vi "Choreo_Choreo_LoadTrajectoryType.vi"(11 "FileName":string="C:\\Users\\Jim\\Desktop\\PathPlanner24\\Choreo\\ChoreoTest.TRAJ") -> (0 "error out":errorcluster, 3 "TrajectoryType":T1, 4 "Full Filename":string)   [LabVIEW 2019, in "ChoreoLib.lvlib"]
doc: "Determine the type of trajectory of a file in the deploy directory. Choreolib expects .traj files to be placed in /deploy/choreo/<trajectoryName>.traj.\n\nInputs: \n - filename - string - The name of the trajectory file. See notes below on file naming.\n\nOutputs:\n - TrajectoryType - enum - Type of trajectory found in the file.\n - Error out - cluster - Error cluster\n - Full Filename - string - fully qualified file name.\n\nNotes on file naming:\n - The file does not need to include the \".traj\" extension. This is added if not present.\n - The file name can be a simple file or an absolute path. If a simple file name is used the default path on the RoboRIO is: \"home:\\lvuser\\natinst\\LabVIEW Data\\choreo\". On a Windows PC the default path is the LabVIEW default directory\\choreo. Normally this is: “%HOMEDRIVE%%HOMEPATH%\\Documents\\LabView Data\\choreo\".\n - Filenames on the RoboRIO, which runs Linux, are case sensitive."
uses:
  ChoreoLib.lvlib
  ENum/Choreo_Util_TrajectoryType.ctl
panel:
  in  "error in (no error)":errorcluster
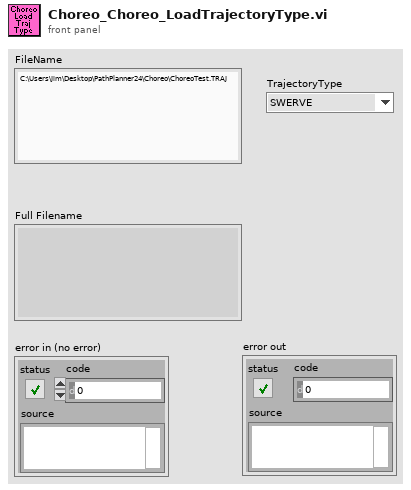
[diagram p1: front panel]
types:
  T1 = typedef "ChoreoLib.lvlib/Choreo_Util_TrajectoryType.ctl" = enum16{"SWERVE", "DIFFERENTIAL", "UNKNOWN"}
  T2 = enum16{"open", "replace", "create", "open or create", "replace or create", "replace or create with confirmation"}
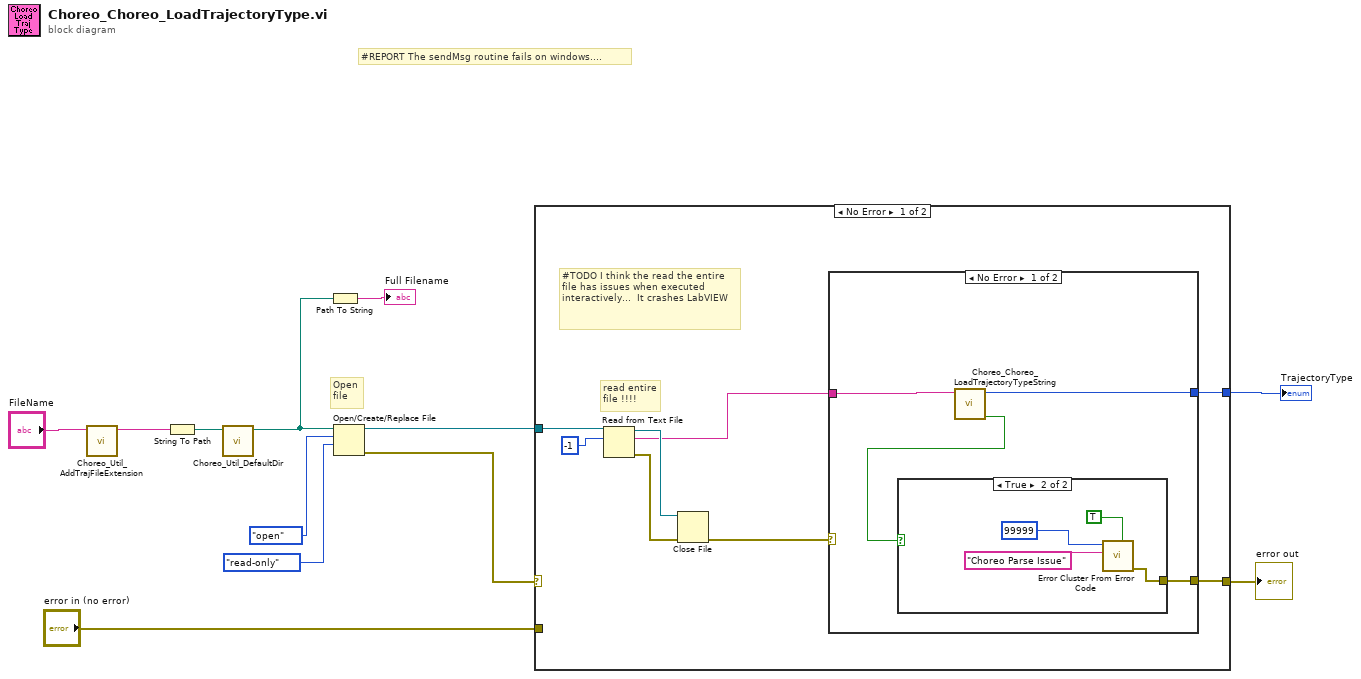
[diagram p0: block diagram]
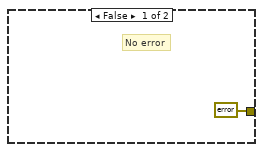
[diagram p2: hidden frame]
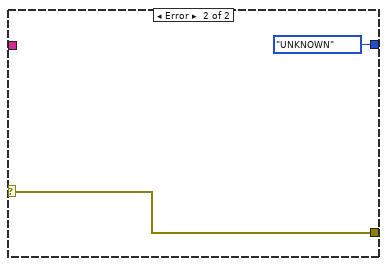
[diagram p3: hidden frame]
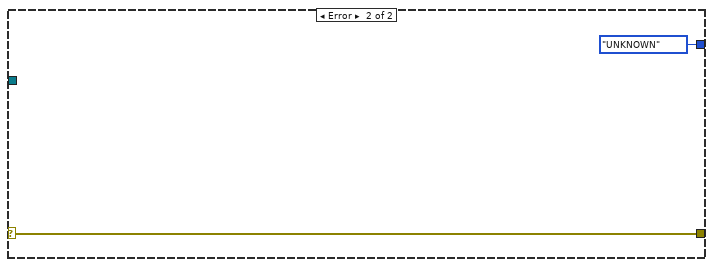
[diagram p4: hidden frame]
diagram:
  # "#REPORT The sendMsg routine fails on windows...."
  # "Open\nfile"
  n1 = call "Choreo_Util_AddTrajFileExtension.vi"("FileName in"="FileName") -> ("FileName out"=w2:string)  [unwired: 10 in]
  n2 = String To Path(string=w2) -> (path=w5:path)
  n3 = call "Choreo_Util_DefaultDir.vi"("Path in"=w5) -> ("Path Out"=w4:path)  [unwired: 10 in]
  n4 = Path To String(path=w4) -> (string=→"Full Filename":string)
  n5 = Open/Create/Replace File(file path (use dialog)=w4, operation (0:open)=T2."open", access (0:read/write)=enum16{"read/write", "read-only", "write-only"}."read-only") -> (refnum out=w8:refnum<file>, error out=w10:errorcluster)  [unwired: 3 in, 1 out]
  n6 = case shown="No Error" w10 {
    selector: w10 -> [_ w33]
    tunnel: w8 -> [w19 _]
    tunnel: [w14 w33] -> w6
    tunnel: "error in (no error)" -> [_ _]
    tunnel: [w13 Choreo_Util_TrajectoryType."UNKNOWN" ("TrajectoryType")] -> w3
    frame No Error {
      # "#TODO I think the read the entire\nfile has issues when executed\ninteractively...  It crashes LabVIEW"
      # "read entire\nfile !!!!"
      n7 = Read from Text File(file (use dialog)=w19, count=-1) -> (refnum out=w18:refnum<file>, text=w17:string, error out=w16:errorcluster)  [unwired: 2 in, 1 out]
      n8 = Close File(refnum=w18, error in=w16) -> (error out=w15:errorcluster)  [unwired: 1 out]
      n9 = case shown="No Error" w15 {
        selector: w15 -> [_ w31]
        tunnel: w17 -> [w23 _]
        tunnel: [w24 w31] -> w14
        tunnel: [w21 Choreo_Util_TrajectoryType."UNKNOWN" ("TrajectoryType")] -> w13
        frame No Error {
          n10 = call "Choreo_Choreo_LoadTrajectoryTypeString.vi"("trajectoryJsonString"=w23) -> ("Error"=w22:bool, "TrajectoryType"=w21:T1)  [unwired: 9 in]
          n11 = case shown="True" w22 {
            tunnel: [errorcluster {"status"=FALSE, "code"=0, "source"=""} ("error out") w26] -> w24
            frame False {
              # "No error"
            }
            frame True {
              n12 = call <vilib>:"Error Cluster From Error Code.vi"("is warning? (False)"=TRUE, "error message (\"\")"="Choreo Parse Issue" ("error message (\"\")"), "error code (0)"=99999) -> ("error out"=w26:errorcluster)  [unwired: 6 in]
            }
          }
        }
        frame Error {
        }
      }
    }
    frame Error {
    }
  }
  "error out" <- w6
  "TrajectoryType" <- w3
